vi "NI PXI-4110 Programmable Power Supply RT Driver VI.vi"(6 "Device Clock":string, 9 "Device Inputs FIFO":refnum<k33>, 11 "Device Reference":T1 format="%.0x") -> ()   [LabVIEW 2015, in "NI PXI-4110 Programmable Power Supply Custom Device.lvlib"]
uses:
  NI PXI-4110 Programmable Power Supply Custom Device.lvlib
  <vilib>/NI Veristand/Custom Device API/Custom Device Item Ref.ctl
  <vilib>/NI Veristand/Custom Device API/Custom Device Channel Type.ctl
  <vilib>/Platform/TimedLoop/XDataNode/timing_clust.ctl
  <vilib>/Platform/TimedLoop/XDataNode/nitl_modes.ctl
  <vilib>/Platform/TimedLoop/XDataNode/wakeup.ctl
  <vilib>/Platform/TimedLoop/XDataNode/XDataNode.xnode
  <vilib>/Platform/TimedLoop/XDataNode/XDNodeRunTimeDep.lvlib
  <vilib>/NI VeriStand/Custom Device API/Custom Device API.lvlib
  <vilib>/NI Veristand/Custom Device Tools/Custom Device Utility Library/Custom Device Utility Library.lvlib
panel:
  in  "Status Notifier":refnum<notifier>
  # "Custom Device Template\nv1.0"
  # "Use this template as a starting point for creating a custom device code module. The input controls shown here are specially named controls that the system will use to provide the device loop with data. The controls are not required for the device loop to run. For instance, if the device doesn't produce any output data, then you don't need the Device Outputs FIFO control. If you do use these controls, however, they need to have these exact names to be functional."
  # "The optional status notifier element is used to notify the RT engine of the last state of the custom device, and to indicate the device has completed execution. If this control is not used, a default No Error value is returned to the system when the device finishes execution.\n\nNote: This error state is not checked until the system shuts down. Use an output status channel to send more immediate status values to the system."
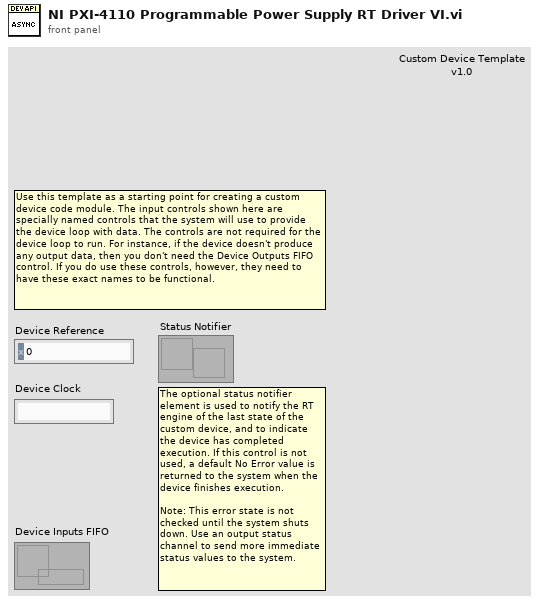
[diagram p1: front panel]
types:
  T1 = typedef "Custom Device API.lvlib/Custom Device Item Ref.ctl" = u64
  T2 = typedef "Custom Device API.lvlib/Custom Device Channel Type.ctl" = enum16{"Input", "Output"}
  T3 = typedef "Custom Device API.lvlib/Custom Device Timed Loop Priority.ctl" = enum32{"Low", "Medium", "High"}
  T4 = cluster{"instrument handle out":refnum<k15>, "Value":string, "Value":u16}[]
  T5 = typedef "XDNodeRunTimeDep.lvlib/timing_clust.ctl" = cluster{"Expected End [f-1]":u64, "Actual End [f-1]":u64, "Finished Late? [f-1]":bool, "Expected End [i-1]":u64, "Actual End [i-1]":u64, "Finished Late? [i-1]":bool, "Expected Start [i]":u64, "Actual Start [i]":u64, "Expected Start [f]":u64, "Actual Start [f]":u64, "Source Name":string, "Structure Name":string, "Period":i64, "Deadline":i64, "Offset":i64, "Start":i64, "Priority":i32, "Timeout":i32, "Mode":T6, "Wakeup Reason":T7, "Error":errorcluster, "Source Type":string, "Secondary Source Type":string, "Global End Time":u64, "Global Start Time":u64, "Frame Duration":u64, "Iteration Duration":u64, "Assigned CPU":i32, "I/O Scan Engine Mode":u32}
  T6 = typedef "XDNodeRunTimeDep.lvlib/nitl_modes.ctl" = enum32{"No Change", "Process missed periods, maintain original phase", "Discard missed periods, maintain original phase", "Process missed periods, ignore original phase", "Discard missed periods, ignore original phase"}
  T7 = typedef "XDNodeRunTimeDep.lvlib/wakeup.ctl" = enum32{"Normal", "Aborted", "Asynchronous wakeup", "Timing source error", "Timed loop error", "Timeout"}
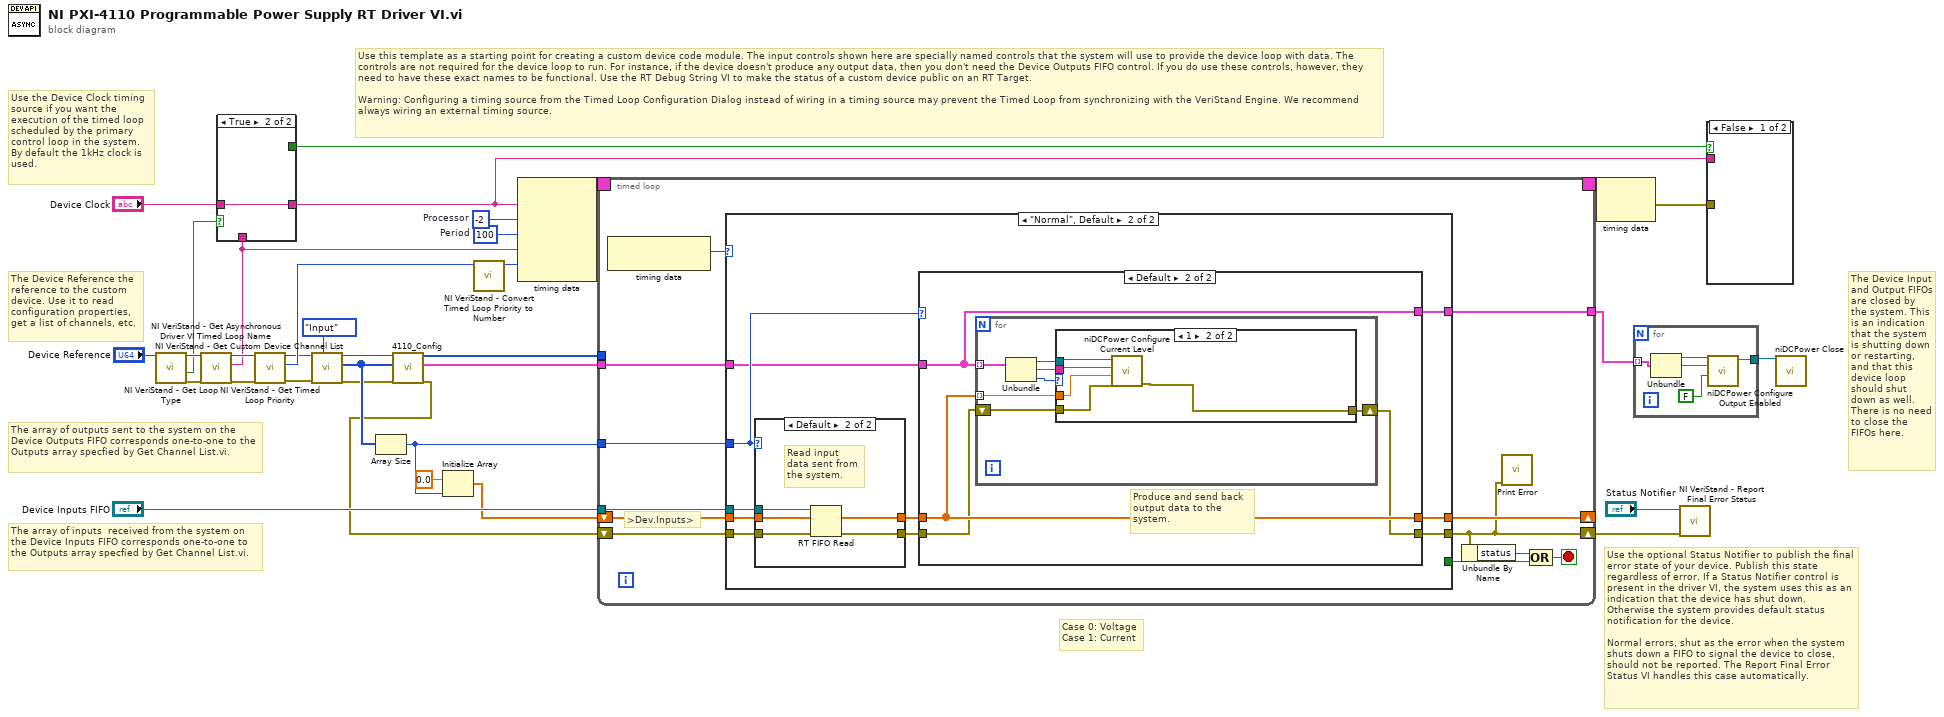
[diagram p0: block diagram]
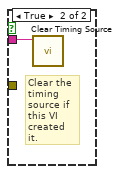
[diagram p2: hidden frame]
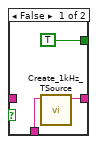
[diagram p3: hidden frame]
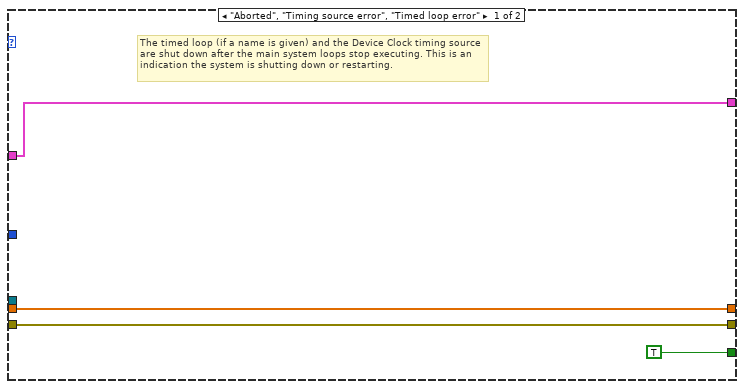
[diagram p4: hidden frame]
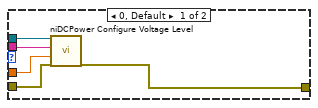
[diagram p6: hidden frame]
diagram:
  w24 = i64 100  # Period
  w25 = -2  # Processor
  # "Case 0: Voltage\nCase 1: Current"
  # "The array of inputs  received from the system on the Device Inputs FIFO corresponds one-to-one to the Outputs array specfied by Get Channel List.vi."
  # "Use the optional Status Notifier to publish the final error state of your device. Publish this state regardless of error. If a Status Notifier control is present in the driver VI, the system uses this as an indication that the device has shut down. Otherwise the system provides default status notification for the device.\n\nNormal errors, shut as the error when the system shuts down a FIFO to signal the device to close, should not be reported. The Report Final Error Status VI handles this case automatically."
  # "The Device Input and Output FIFOs are closed by the system. This is an indication that the system is shutting down or restarting, and that this device loop should shut down as well. There is no need to close the FIFOs here."
  # "The array of outputs sent to the system on the Device Outputs FIFO corresponds one-to-one to the Outputs array specfied by Get Channel List.vi."
  # "The Device Reference the reference to the custom device. Use it to read configuration properties, get a list of channels, etc."
  # "Use the Device Clock timing source if you want the execution of the timed loop scheduled by the primary control loop in the system. \nBy default the 1kHz clock is used."
  # "Use this template as a starting point for creating a custom device code module. The input controls shown here are specially named controls that the system will use to provide the device loop with data. The controls are not required for the device loop to run. For instance, if the device doesn't produce any output data, then you don't need the Device Outputs FIFO control. If you do use these controls, however, they need to have these exact names to be functional. Use the RT Debug String VI to make the status of a custom device public on an RT Target.\n\nWarning: Configuring a timing source from the Timed Loop Configuration Dialog instead of wiring in a timing source may prevent the Timed Loop from synchronizing with the VeriStand Engine. We recommend always wiring an external timing source."
  n1 = call <vilib>:"NI VeriStand - Get Loop Type.vi"("Device Ref in"="Device Reference") -> ("error out"=w23:errorcluster, "Use Device Clock"=w20:bool, "Device Ref out"=w22:T1)  [unwired: 1 in, 7 out]
  n2 = call <vilib>:"NI VeriStand - Get Asynchronous Driver VI Timed Loop Name.vi"("error in (no error)"=w23, "Device Ref in"=w22) -> ("error out"=w28:errorcluster, "Device Timed Loop Name"=w14:string, "Device Ref out"=w34:T1)  [unwired: 7 out]
  n3 = case shown="True" w20 {
    tunnel: "Device Clock" -> [_ w38]
    tunnel: [w37 w38] -> w15
    tunnel: [TRUE _] -> w16
    tunnel: w14 -> [w35 _]
    frame False {
      n4 = call <vilib>:"Create_1kHz_TSource.vi"("name (in)"=w35) -> ("name (out)"=w37:string)  [unwired: 1 in, 9 out]
    }
    frame True {
    }
  }
  n5 = call <vilib>:"NI VeriStand - Get Timed Loop Priority.vi"("error in (no error)"=w28, "Device Ref in"=w34) -> ("error out"=w1:errorcluster, "Priority"=w27:T3, "Device Ref out"=w13:T1)  [unwired: 7 out]
  n6 = call <vilib>:"NI VeriStand - Get Custom Device Channel List.vi"("Channel Type"=Custom_Device_Channel_Type."Input", "error in (no error)"=w1, "Device Ref in"=w13) -> ("error out"=w9:errorcluster, "Specified Channel Ref List"=w10:T1[], "Device Ref out"=w12:T1)  [unwired: 6 out]
  n7 = Array Size(array=w10) -> (size(s)=w3:i32)
  n8 = call "4110_Config.vi"("error in (no error)"=w9, "Specified Channel Ref List"=w10, "Device Ref out"=w12) -> ("error out"=w2:errorcluster, "Channel Info"=w8:T4, "Channel Ref List (out)"=w11:T1[])  [unwired: 6 in]
  n9 = Initialize Array(0.0 ("element"), w3) -> (w29:dbl[])
  n10 = call <vilib>:"NI VeriStand - Convert Timed Loop Priority to Number.vi"("Priority"=w27) -> ("Numeric Priority"=w26:i32)  [unwired: 10 out]
  n11 = node-c288(w15, w25, w24, w14, w26) -> (w32:T5)
  n12 = timed-loop {
    timing: w32 -> [_]
    timing-out: [_] -> w31
    shift-right: [w48] -> _
    shift-left: w29 -> [w49]
    shift-right: [w39] -> w6
    shift-left: w2 -> [w50]
    tunnel: "Device Inputs FIFO" -> [w46]
    tunnel: w3 -> [w42]
    tunnel: w11 -> [_]
    tunnel: w8 -> [w41]
    tunnel: [w40] -> w7
    stop <- w43 stop-if-true
    # ">Dev.Inputs>"
    n13 = node-c288() -> (w47:T7)  [unwired: 1 out]
    n14 = case shown="\"Normal\", Default" w47 {
      tunnel: w50 -> [w53 w59]
      tunnel: w49 -> [w54 w63]
      tunnel: [w53 w60] -> w39
      tunnel: [w54 w58] -> w48
      tunnel: w46 -> [_ w64]
      tunnel: [TRUE _] -> w44
      tunnel: w42 -> [_ w57]
      tunnel: w41 -> [w51 w56]
      tunnel: [w51 w55] -> w40
      frame "Aborted", "Timing source error", "Timed loop error" {
        # "The timed loop (if a name is given) and the Device Clock timing source are shut down after the main system loops stop executing. This is an indication the system is shutting down or restarting."
      }
      frame "Normal", Default {
        n15 = case shown="Default" w57 {
          tunnel: w64 -> [_ w95]
          tunnel: w63 -> [w90 w94]
          tunnel: [w90 w93] -> w62
          tunnel: [w89 w92] -> w61
          tunnel: w59 -> [w89 w91]
          frame 0 {
            # "No inputs to read\nfrom system. Inputs FIFO not created in this case, so don't write to it."
          }
          frame Default {
            # "Read input data sent from the system."
            n16 = RT FIFO Read(0:w95, 1:w94, 3:w91) -> (9:w93:dbl[], 11:w92:errorcluster)  [unwired: 4 out]
          }
        }
        n17 = case shown="Default" w57 {
          tunnel: w62 -> [w67 w71]
          tunnel: w61 -> [w66 w70]
          tunnel: [w66 w69] -> w60
          tunnel: [w67 w71] -> w58
          tunnel: w56 -> [w65 w68]
          tunnel: [w65 w68] -> w55
          frame 0 {
            # "No outputs to write to system. The Device Outputs FIFO is never created in this case, so don't write to it."
          }
          frame Default {
            # "Produce and send back output data to the system."
            n18 = for {
              tunnel: w68 -> [w78] mode=indexing
              tunnel: w71 -> [w72] mode=indexing
              shift-right: [w74] -> w69
              shift-left: w70 -> [w75]
              n19 = Unbundle(w78) -> ("instrument handle out"=w77:refnum<k15>, "Value"=w76:string, "Value"=w73:u16)
              n20 = case shown="1" w73 {
                tunnel: w77 -> [w83 w88]
                tunnel: w76 -> [w80 w86]
                tunnel: w72 -> [w82 w85]
                tunnel: w75 -> [w81 w87]
                tunnel: [w79 w84] -> w74
                frame 0, Default {
                  n21 = call <instrlib>:"niDCPower Configure Voltage Level.vi"("error in (no error)"=w81, "voltage level"=w82, "channel name"=w80, "instrument handle"=w83) -> ("error out"=w79:errorcluster)  [unwired: 6 in, 1 out]
                }
                frame 1 {
                  n22 = call <instrlib>:"niDCPower Configure Current Level.vi"("error in (no error)"=w87, "current level"=w85, "channel name"=w86, "instrument handle"=w88) -> ("error out"=w84:errorcluster)  [unwired: 6 in, 1 out]
                }
              }
            }
          }
        }
      }
    }
    n23 = Unbundle By Name(w39) -> ("status"=w45:bool)
    n24 = call "Print Error.vi"("error out"=w39) -> ()  [unwired: 10 in]
    n25 = Compound Arithmetic op=OR(w45, w44) -> (w43:bool)
  }
  n26 = node-c288(w31) -> (w17:errorcluster)
  n27 = for {
    tunnel: w7 -> [w103] mode=indexing
    tunnel: [w99] -> w4
    n28 = Unbundle(w103) -> ("instrument handle out"=w102:refnum<k15>, "Value"=w101:string)  [unwired: 1 out]
    n29 = call <instrlib>:"niDCPower Configure Output Enabled.vi"("output enabled"=FALSE, "channel name"=w101, "instrument handle"=w102) -> ("instrument handle out"=w99:refnum<k15>)  [unwired: 7 in, 1 out]
  }
  n30 = call <vilib>:"NI VeriStand - Report Final Error Status.vi"("error in (no error)"=w6, "Status Notifier"="Status Notifier") -> ()  [unwired: 1 in, 9 out]
  n31 = case shown="False" w16 {
    tunnel: w17 -> [_ _]
    tunnel: w15 -> [_ w104]
    frame False {
    }
    frame True {
      # "Clear the timing source if this VI created it."
      n32 = call <vilib>:"Clear Timing Source.vi"("name"=w104) -> ()  [unwired: 1 in, 10 out]
    }
  }
  n33 = call <instrlib>:"niDCPower Close.vi"("instrument handle"=w4) -> ()  [unwired: 10 in, 1 out]
